vi "Write Collection.vi"(8 "error in (no error)":errorcluster, 10 "Collection":refnum<class "Test Runner.lvclass">[](array[class]), 11 "Test Runner.Collection in":refnum<class "Test Runner.Collection.lvclass">) -> (0 "error out":errorcluster, 3 "Test Runner.Collection out":refnum<class "Test Runner.Collection.lvclass">)   [LabVIEW 2013, in "Caraya.lvlib" / "Test Runner.Collection.lvclass"]
uses:
  Test Runner.Collection.lvclass
  Test Runner/Test Runner.lvclass
  Test Runner.Collection.lvclass/Test Runner.Collection.ctl
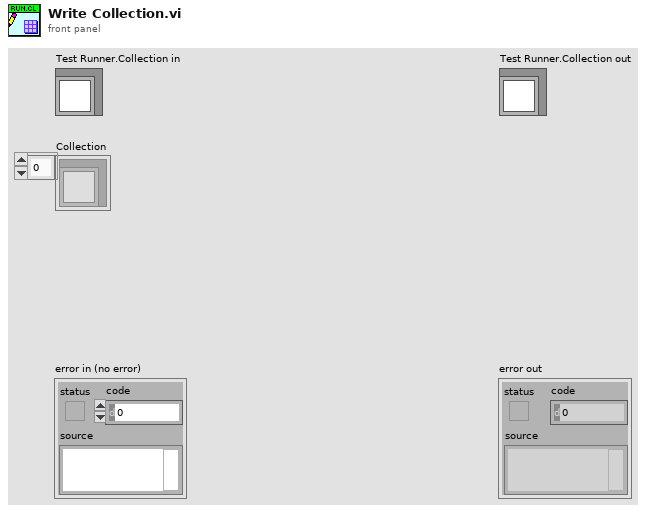
[diagram p1: front panel]
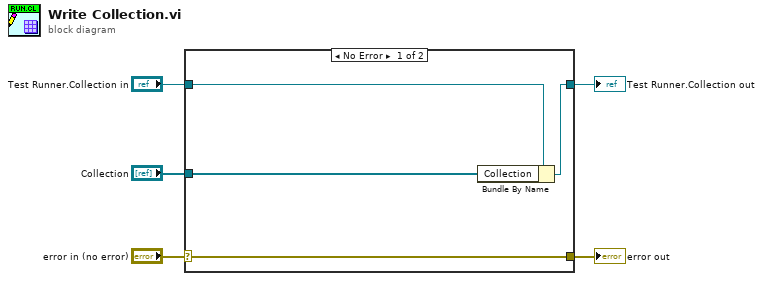
[diagram p0: block diagram]
diagram:
  n1 = case shown="No Error" "error in (no error)" {
    selector: "error in (no error)" -> [w9 w10]
    tunnel: [w9 w10] -> w4
    tunnel: [w7 w11] -> w2
    tunnel: "Test Runner.Collection in" -> [w8 w11]
    tunnel: "Collection" -> [w6 _]
    frame No Error {
      n2 = Bundle By Name(cluster=w8, "Collection"=w6) -> (w7:refnum<class "Test Runner.Collection.lvclass">)
    }
    frame Error {
    }
  }
  "error out" <- w4
  "Test Runner.Collection out" <- w2
